vi "Write Acoustic Calibration File.vi"(0 "Cal File Path":path, 5 "Per Site Acoustic Cal Data":T1[](array[typedef]), 11 "error in (no error)":errorcluster) -> (15 "error out":errorcluster)   [LabVIEW 2020]
doc: "Write Acoustic Calibration API writes the input calibration data for each site into the calibration file path passed as inputs."
uses:
  Acoustic Cal Data Cluster.ctl
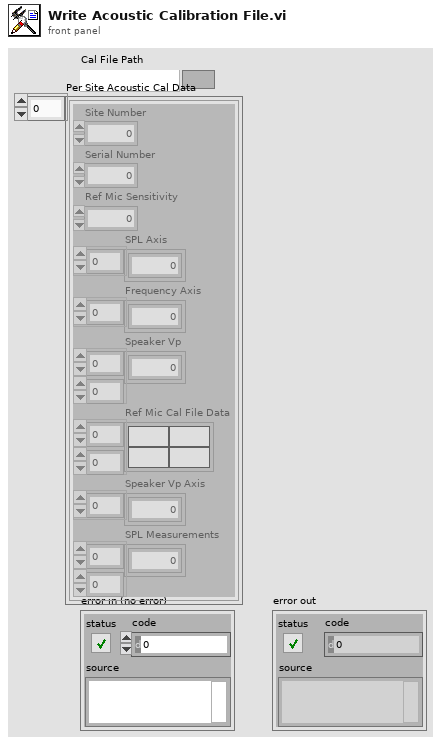
[diagram p1: front panel]
types:
  T1 = typedef "Acoustic Cal Data Cluster.ctl" = cluster{"Site Number":i32, "Serial Number":u32, "Ref Mic Sensitivity":dbl, "SPL Axis":dbl[], "Frequency Axis":dbl[], "Speaker Vp":dbl[][], "Ref Mic Cal File Data":string[][], "Speaker Vp Axis":dbl[], "SPL Measurements":dbl[][]}
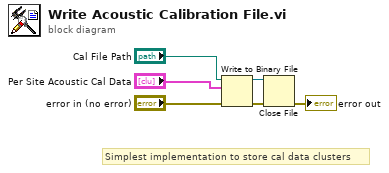
[diagram p0: block diagram]
diagram:
  # "Simplest implementation to store cal data clusters"
  n1 = Write to Binary File(file (use dialog)="Cal File Path", data="Per Site Acoustic Cal Data", error in="error in (no error)") -> (refnum out=w1:refnum<file>, error out=w3:errorcluster)  [unwired: 3 in, 1 out]
  n2 = Close File(refnum=w1, error in=w3) -> (error out=→"error out":errorcluster)  [unwired: 1 out]
